vi "device_init.vi"(10 "Device ID":refnum<vi>, 11 "Serial #":refnum<vi>) -> (0 "error out":errorcluster, 1 ".NET Refnum out":refnum<k24>)   [LabVIEW 2020]
uses:
  C:/Users/359167/Documents/LabVIEW_ws/Thorlabs.MotionControl.DeviceManagerCLI.dll
  359167/Documents/LabVIEW_ws/Thorlabs.MotionControl.DeviceManagerCLI.dll
  C:/Users/359167/Documents/LabVIEW_ws/Thorlabs.MotionControl.KCube.InertialMotorCLI.dll
  359167/Documents/LabVIEW_ws/Thorlabs.MotionControl.KCube.InertialMotorCLI.dll
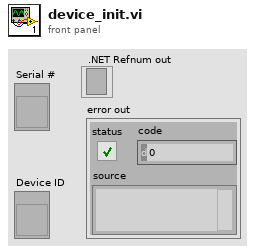
[diagram p1: front panel]
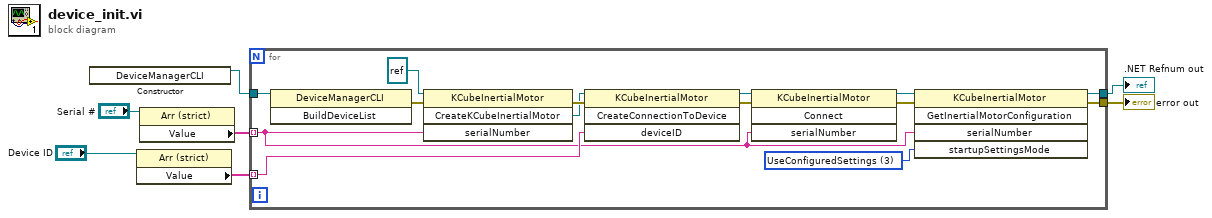
[diagram p0: block diagram]
diagram:
  n1 = constructor class="DeviceManagerCLI" ("Constructor Node")() -> (reference out=w4:refnum<k24>)  [unwired: 3 in, 2 out]
  n2 = property class="Arr (strict)"(reference="Device ID") -> ("Value"=w7:string[])  [unwired: 1 in, 2 out]
  n3 = property on="Property Node" class="Arr (strict)"(reference="Serial #") -> ("Value"=w3:string[])  [unwired: 1 in, 2 out]
  n4 = for {
    tunnel: w3 -> [w8] mode=indexing
    tunnel: w4 -> [w21]
    tunnel: [w10] -> w5
    tunnel: [w9] -> w6
    tunnel: w7 -> [w11] mode=indexing
    w16 = 3 items=["UseDeviceSettings"=1, "UseFileSettings"=2, "UseConfiguredSettings"=3] ("startupSettingsMode")
    n5 = invoke class="DeviceManagerCLI" method="BuildDeviceList"(reference=w21) -> (error out=w19:errorcluster)  [unwired: 2 in, 2 out]
    n6 = invoke class="KCubeInertialMotor" method="CreateKCubeInertialMotor"(reference=refnum<k24> refnum, error in=w19, "serialNumber"=w8) -> (error out=w18:errorcluster, "CreateKCubeInertialMotor"=w17:refnum<k24>)  [unwired: 1 in, 2 out]
    n7 = invoke class="KCubeInertialMotor" method="CreateConnectionToDevice"(reference=w17, error in=w18, "deviceID"=w11) -> (reference out=w15:refnum<k24>, error out=w14:errorcluster)  [unwired: 1 in, 2 out]
    n8 = invoke class="KCubeInertialMotor" method="Connect"(reference=w15, error in=w14, "serialNumber"=w8) -> (reference out=w13:refnum<k24>, error out=w12:errorcluster)  [unwired: 1 in, 2 out]
    n9 = invoke class="KCubeInertialMotor" method="GetInertialMotorConfiguration"(reference=w13, error in=w12, "serialNumber"=w8, "startupSettingsMode"=w16) -> (reference out=w10:refnum<k24>, error out=w9:errorcluster)  [unwired: 1 in, 3 out]
  }
  "error out" <- w6
  ".NET Refnum out" <- w5
